vi "Create Client.vi"(8 "error in":errorcluster, 10 "certificatePath":string, 11 "address":string) -> (0 "error out":errorcluster, 3 "ClientID out":T1)   [LabVIEW 2019, in "grpc-lvsupport.lvlib"]
uses:
  grpc-lvsupport.lvlib
  Shared/grpcId.ctl
  <vilib>/Utility/error.llb/Error Cluster From Error Code.vi
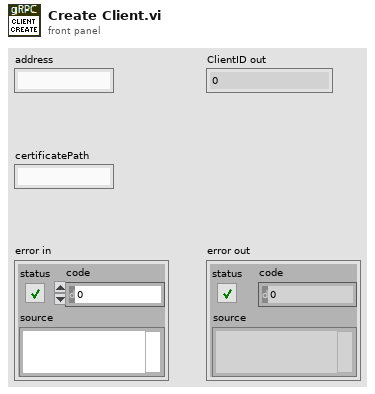
[diagram p1: front panel]
types:
  T1 = typedef "grpc-lvsupport.lvlib/grpcId.ctl" = u64
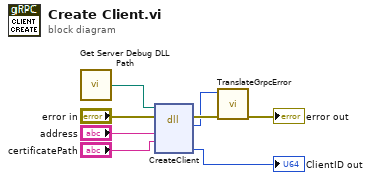
[diagram p0: block diagram]
diagram:
  n1 = call "Get Server Debug DLL Path.vi"() -> ("Server Debug DLL Path"=w6:path)
  n2 = dll-call lib="?" fn="CreateClient"(path in=w6, error in="error in", "address"="address", "certificatePath"="certificatePath") -> (error out=w7:errorcluster, "return type"=w1:i32, "clientId"=→"ClientID out":u64)  [unwired: 4 in, 1 out]
  n3 = call "TranslateGrpcError.vi"("error in"=w7, "Error Code"=w1) -> ("error out"=→"error out":errorcluster)  [unwired: 9 in]
